vi "open all relay channel.vi"(8 "error in (no error)":errorcluster caption="entrée d'erreur (pas d'erreur)", 11 "hHandle":i32) -> (0 "error out":errorcluster caption="sortie d'erreur")   [LabVIEW 2020, in "usb_relay_device.lvlib"]
doc: "int EXPORT_API usb_relay_device_open_all_relay_channel(int hHandle);"
uses:
  usb_relay_device.lvlib
  usb_relay_device.dll
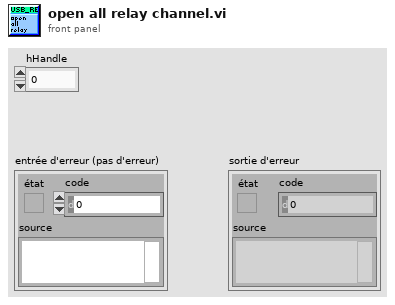
[diagram p1: front panel]
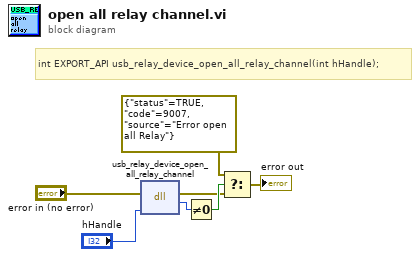
[diagram p0: block diagram]
diagram:
  # "int EXPORT_API usb_relay_device_open_all_relay_channel(int hHandle);"
  n1 = dll-call lib="C:/Users/ngarcin/OneDrive - Altyor/Standard TB/Class/Relay_Board/Relay_Board usb_Relay_device/usb_relay_device/usb_relay_device.*" fn="usb_relay_device_open_all_relay_channel"(error in="error in (no error)", "hHandle"="hHandle") -> (error out=w2:errorcluster, w1:i32)  [unwired: 3 in, 1 out]
  n2 = Not Equal To 0?(x=w1) -> (x != 0?=w5:bool)
  n3 = Select(t=errorcluster {"status"=TRUE, "code"=9007, "source"="Error open all Relay"} ("sortie d'erreur"), s=w5, f=w2) -> (s? t:f=→"error out":errorcluster)
